vi "Untitled 1.vi"() -> ()   [LabVIEW 2019]
uses:
  <vilib>/Instr/_visa.llb/VISA Configure Serial Port (Instr).vi
panel:
  out "message 3":string caption="Result"
  in  "auto button":bool
  in  "inverse fan status button":bool
  out "comment":string
  out "remaining string":string
  out "trimmed string":string
  out "read buffer":string
  out "message 2":string caption="Result"
  in  "Max Temperature":dbl
  out "message 1":string caption="Result"
  in  "Humidty Button":bool
  in  "stop":bool
  in  "Tempurature Button":bool
  in  "Max Humidtiy":dbl
  out "Max Temperature status":bool
  out "Fan status":bool
  out "Humidity Gauge en %":dbl(knob) scale=0.1..100.0
  out "Temperature Gauge en °C":dbl(knob) scale=0.0..50.0
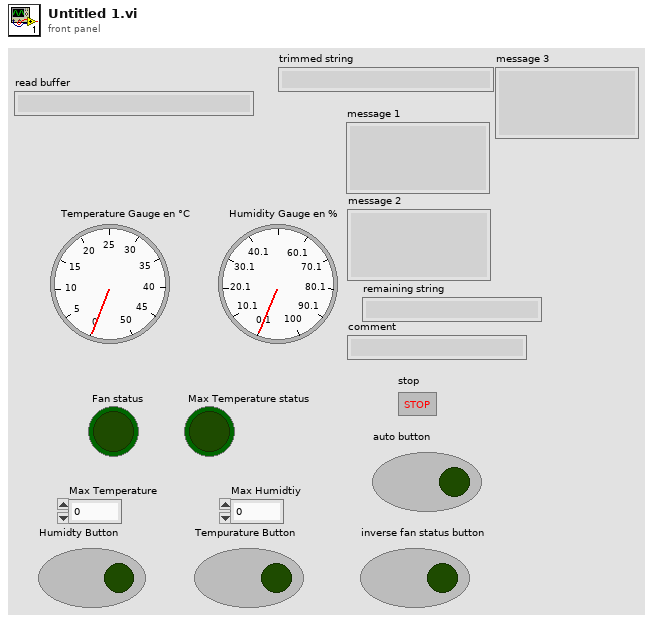
[diagram p1: front panel]
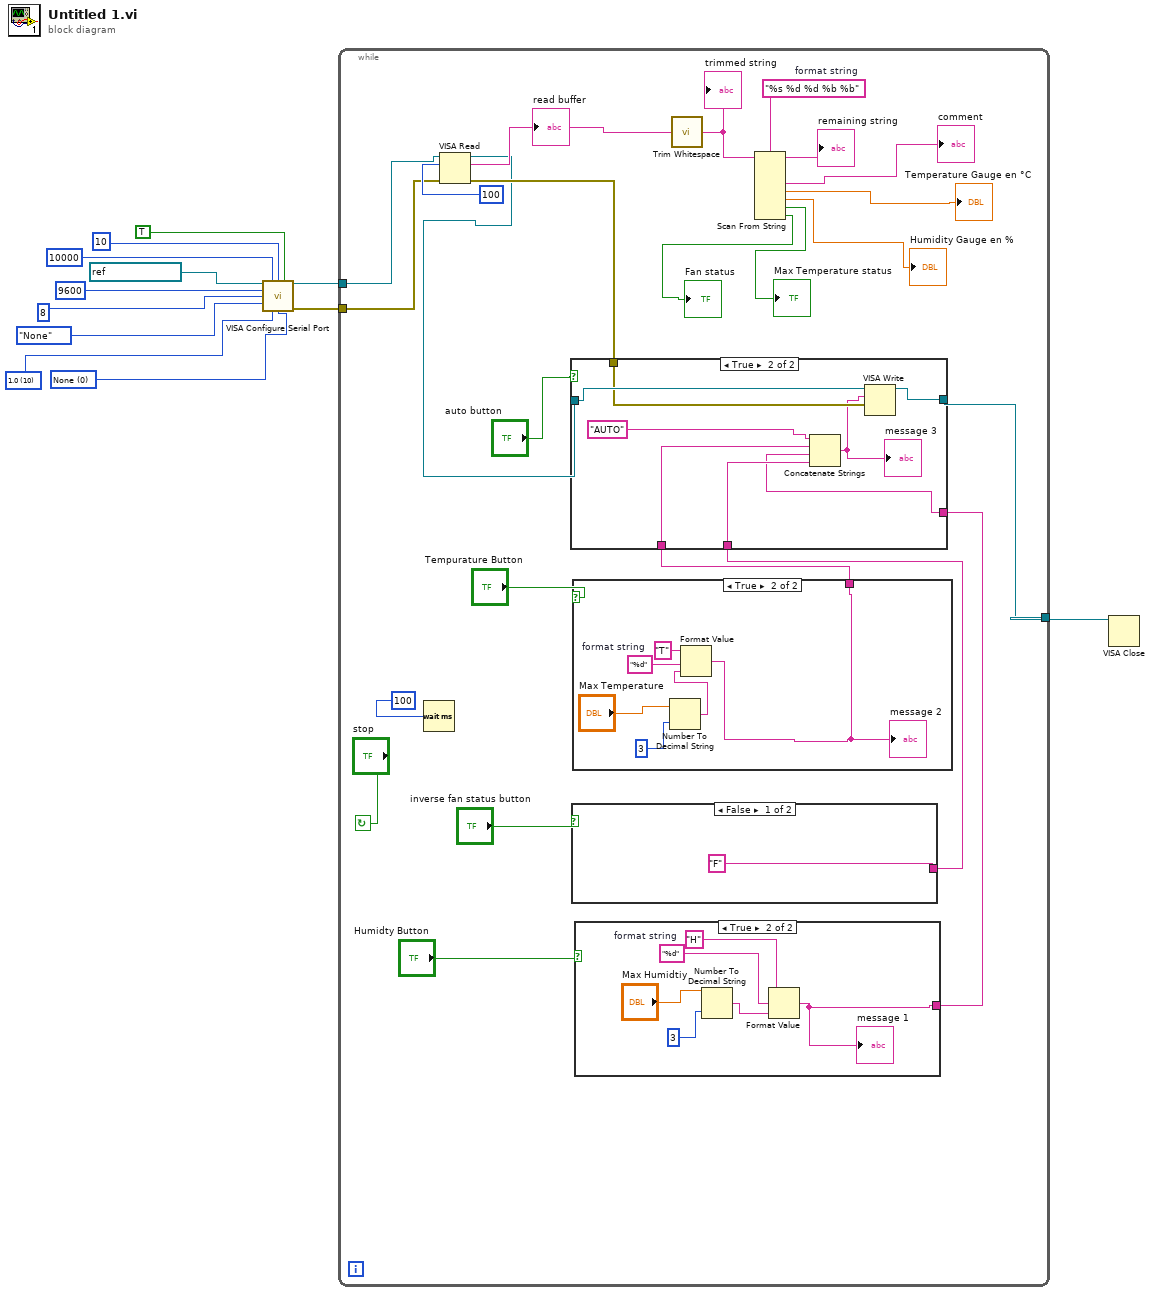
[diagram p0: block diagram]
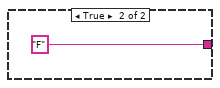
[diagram p3: hidden frame]
diagram:
  w7 = u16 0 items=["None", "XON/XOFF", "RTS/CTS", "XON/XOFF & RTS/CTS", "DTR/DSR", "XON/XOFF & DTR/DSR"] ("flow control (0:none)")
  w8 = u16 10 items=["1.0"=10, "1.5"=15, "2.0"=20] ("stop bits (10: 1 bit)")
  n1 = call-poly "VISA Configure Serial Port"("VISA resource name"=refnum<visa-resource-name> "COM16", "timeout (10sec)"=u32 10000, "termination char\n(0xA = '\\n' = LF)"=u8 10 ("termination char\n(0xA = '\\n' = LF)"), "Enable Termination\nChar (T)"=TRUE ("Enable Termination\nChar (T)"), "baud rate (9600)"=u32 9600, "data bits (8)"=u16 8, "parity (0:none)"=enum16{"None", "Odd", "Even", "Mark", "Space"}."None", "stop bits (10: 1 bit)"=w8, "flow control (0:none)"=w7) -> ("VISA resource name out"=w3:refnum<visa-resource-name>, "error out"=w1:errorcluster)  [unwired: 5 in]
  n2 = while {
    tunnel: w3 -> [w19]
    tunnel: [w18] -> w2
    tunnel: w1 -> [w21]
    stop <- "stop" continue-if-true
    w33 = "%s %d %d %b %b"  # format string
    n3 = Wait (ms)(milliseconds to wait=u32 100) -> ()  [unwired: 1 out]
    n4 = VISA Read(VISA resource name=w19, byte count=u32 100, error in (no error)=w21) -> (read buffer=w32:string, error out=w20:errorcluster)  [unwired: 2 out]
    "read buffer" <- w32
    n5 = case shown="False" "inverse fan status button" {
      tunnel: ["F" ("string (\"\")") "F" ("string (\"\")")] -> w16
      frame False {
      }
      frame True {
      }
    }
    n6 = case shown="True" "Tempurature Button" {
      tunnel: [_ w44] -> w17
      frame False {
      }
      frame True {
        w47 = "%d"  # format string
        n7 = Number To Decimal String(number="Max Temperature", width (-)=i16 3) -> (decimal integer string=w48:string)
        n8 = Format Value(string ("")="T", format string=w47, value (0)=w48) -> (output string=w44:string)
        "message 2" <- w44
      }
    }
    n9 = case shown="True" "Humidty Button" {
      tunnel: [_ w36] -> w15
      frame False {
      }
      frame True {
        w39 = "%d"  # format string
        n10 = Number To Decimal String(number="Max Humidtiy", width (-)=i16 3) -> (decimal integer string=w40:string)
        n11 = Format Value(string ("")="H", format string=w39, value (0)=w40) -> (output string=w36:string)
        "message 1" <- w36
      }
    }
    n12 = case shown="True" "auto button" {
      tunnel: w19 -> [_ w57]
      tunnel: [_ w56] -> w18
      tunnel: w20 -> [_ w55]
      tunnel: w17 -> [_ w53]
      tunnel: w16 -> [_ w52]
      tunnel: w15 -> [_ w51]
      frame False {
      }
      frame True {
        n13 = Concatenate Strings("AUTO" ("string (\"\")"), w53, w51, w52) -> (w50:string)
        "message 3" <- w50
        n14 = VISA Write(VISA resource name=w57, write buffer=w50, error in (no error)=w55) -> (VISA resource name out=w56:refnum<visa-resource-name>)  [unwired: 2 out]
      }
    }
    n15 = call <vilib>:"Trim Whitespace.vi"("string"=w32) -> ("trimmed string"=w31:string)  [unwired: 1 in]
    "trimmed string" <- w31
    n16 = Scan From String "Scan From String"(format string=w33, input string=w31) -> (remaining string=→"remaining string":string, output 1=→"comment":string, output 2=→"Temperature Gauge en °C":dbl, output 3=→"Humidity Gauge en %":dbl, output 4=→"Max Temperature status":bool, output 5=→"Fan status":bool)  [unwired: 7 in, 2 out]
  }
  n17 = VISA Close(VISA resource name=w2) -> ()  [unwired: 1 in, 1 out]
